vi "test query_components.vi"() -> ()   [LabVIEW 2017]
uses:
  DB Component.ctl
  Database.lvlib
panel:
  in  "part":string
  out "Components":T1[](array[typedef])
  out "error out":errorcluster
  in  "port":i32=33060
  in  "host":string="localhost"
  in  "password":string="carriker"
  in  "username":string="root"
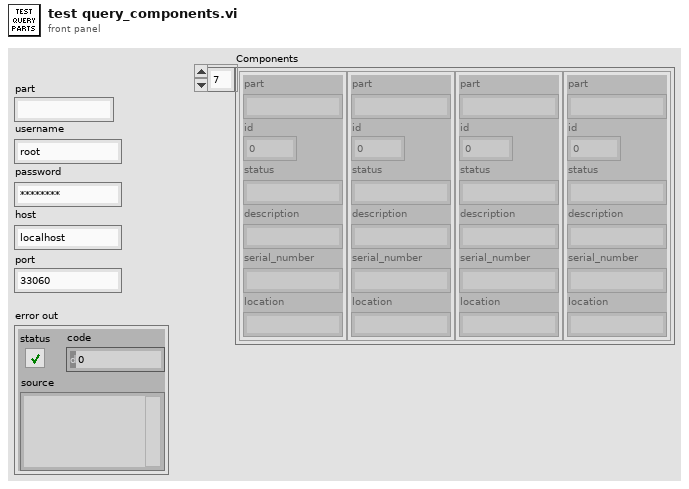
[diagram p1: front panel]
types:
  T1 = typedef "Database.lvlib/DB Component.ctl" = cluster{"part":string, "id":i32, "status":string, "description":string, "serial_number":string, "location":string}
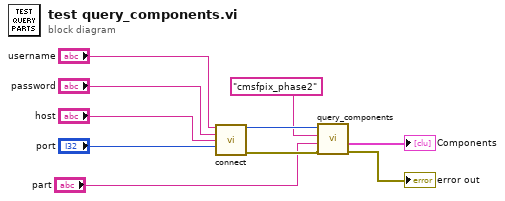
[diagram p0: block diagram]
diagram:
  n1 = call "connect.vi"("username"="username", "password"="password", "host"="host", "port"="port") -> ("DB Session ID"=w6:i32, "error out"=w4:errorcluster)  [unwired: 10 in]
  n2 = call "query_components.vi"("error in (no error)"=w4, "part"="part", "Schema"="cmsfpix_phase2", "DB Session ID"=w6) -> ("error out"=→"error out":errorcluster, "Components"=→"Components":T1[])  [unwired: 4 in, 2 out]
